vi "Complex FFT PtByPt.vi"(2 "initialize":bool, 3 "sample length":i32=100, 5 "x":cdb format="%#.6g") -> (0 "error":i32, 1 "FFT{X}":cdb[](array[numeric]))   [LabVIEW 2017, in "NI_PtbyPt.lvlib"]
doc: "Computes the Fourier transform of <B>x</B>. This VI is similar to the FFT VI. Wire data to the <B>x</B> input to determine the polymorphic instance to use or manually select the instance."
uses:
  <vilib>/ptbypt/NI_PtbyPt.lvlib
  <vilib>/Analysis/1siggen.llb/Ramp Pattern by Samples.vi
  <vilib>/Analysis/NI_AALBase.lvlib
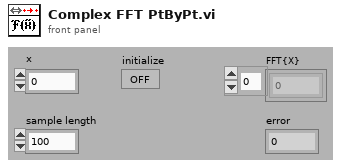
[diagram p1: front panel]
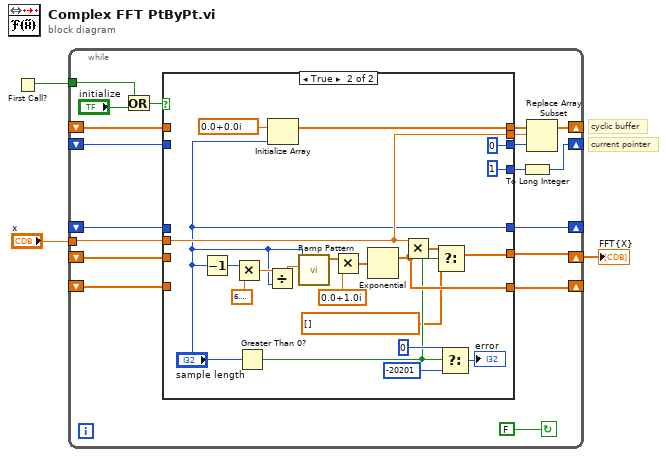
[diagram p0: block diagram]
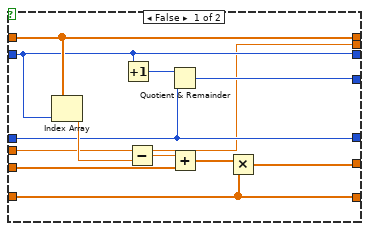
[diagram p2: hidden frame]
diagram:
  # "current pointer"
  # "cyclic buffer"
  n1 = First Call?() -> (First Call?: T/F=w1:bool)
  n2 = while {
    tunnel: w1 -> [w4]
    shift-left: _ -> [w10]
    shift-right: [w11] -> _
    shift-left: _ -> [w13]
    shift-right: [w12] -> _
    shift-left: _ -> [w18]
    shift-right: [w19] -> _
    tunnel: "x" -> [w9]
    shift-left: _ -> [w20]
    shift-right: [w22] -> w2
    shift-left: _ -> [w21]
    shift-right: [w16] -> _
    stop <- FALSE continue-if-true
    n3 = Or(x=w4, y="initialize") -> (x .or. y?=w5:bool)
    n4 = case shown="True" w5 {
      tunnel: w10 -> [w24 _]
      tunnel: [w28 w36] -> w22
      tunnel: [w34 w54] -> w17
      tunnel: w21 -> [w34 _]
      tunnel: w20 -> [w31 _]
      tunnel: [w29 w44] -> w19
      tunnel: w18 -> [w29 _]
      tunnel: [w32 0 ("Index")] -> w15
      tunnel: [w25 1 ("Index")] -> w14
      tunnel: w13 -> [w32 _]
      tunnel: [w24 "sample length"] -> w11
      tunnel: w9 -> [w23 w43]
      tunnel: [w23 w43] -> w8
      frame False {
        n5 = Index Array(array=w34, index=w32) -> (element=w33:cdb)
        n6 = Increment(x=w32) -> (x+1=w26:i32)
        n7 = Subtract(x=w23, y=w33) -> (x-y=w27:cdb)
        n8 = Quotient & Remainder(x=w26, y=w24) -> (x-y*floor(x/y)=w25:i32)  [unwired: 1 out]
        n9 = Add(x=w27, y=w31) -> (x+y=w30:cdb[])
        n10 = Multiply(x=w30, y=w29) -> (x*y=w28:cdb[])
      }
      frame True {
        n11 = Decrement(x="sample length") -> (x-1=w50:i32)
        n12 = Multiply(x=w50, y=6.283185307179586) -> (x*y=w49:dbl)
        n13 = Greater Than 0?(x="sample length") -> (x > 0?=w37:bool)
        n14 = Divide(x=w49, y="sample length") -> (x/y=w48:dbl)
        n15 = Initialize Array(cdb 0.0+0.0i ("Element Data"), "sample length") -> (w54:cdb[])
        n16 = call-poly <vilib>:"Ramp Pattern.vi"("end"=w48, "samples"="sample length") -> ("Ramp Pattern"=w51:dbl[])  [unwired: 8 in, 1 out]
        n17 = Multiply(x=w51, y=cdb 0.0+1.0i) -> (x*y=w45:cdb[])
        n18 = Exponential(1:w45) -> (0:w44:cdb[])
        n19 = Multiply(x=w43, y=w44) -> (x*y=w38:cdb[])
        n20 = Select(t=w38, s=w37, f=cdb[] []) -> (s? t:f=w36:cdb[])
        n21 = Select(t=0, s=w37, f=-20201) -> (s? t:f=→"error":i32)
      }
    }
    n22 = To Long Integer(number=w14) -> (32bit integer=w12:i32)
    n23 = Replace Array Subset(array=w17, new element=w8, index=w15) -> (w16:cdb[])
  }
  "FFT{X}" <- w2
